vi "GaGe4_QueryStatus.vi"(8 "error in (no error)":errorcluster, 11 "Handle Cluster":T1) -> (0 "error out":errorcluster, 1 "Error?":bool, 2 "Triggered":bool, 4 "Complete":bool, 5 "Armed":bool, 6 "Status":string)   [LabVIEW 2015]
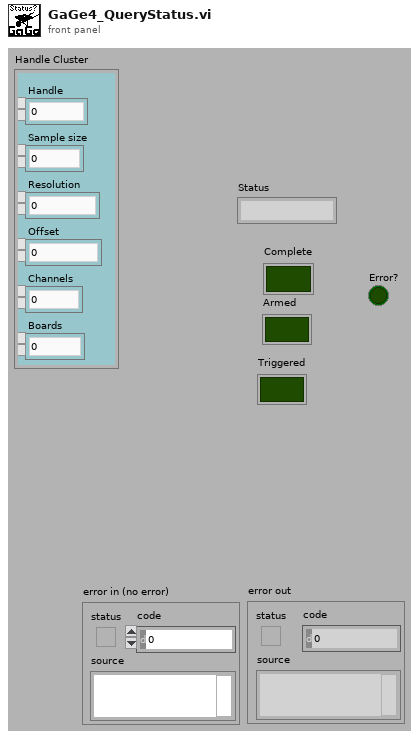
[diagram p1: front panel]
types:
  T1 = cluster{"Handle":u32, "Sample size":u32, "Resolution":i32, "Offset":i32, "Channels":u32, "Boards":u32}
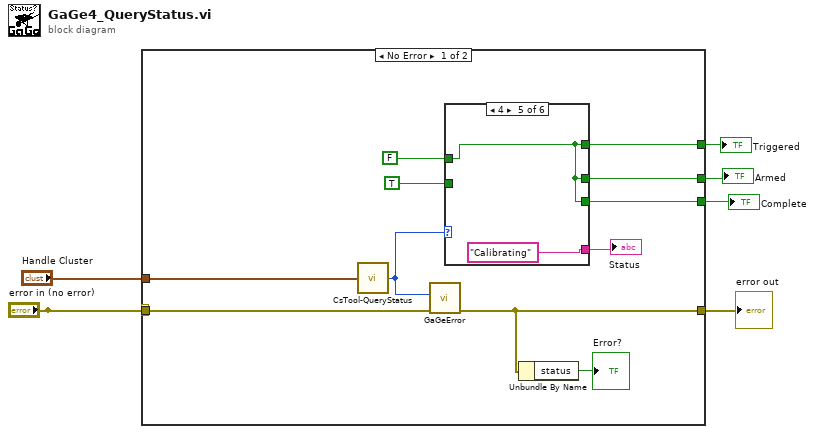
[diagram p0: block diagram]
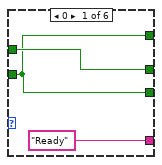
[diagram p2: hidden frame]
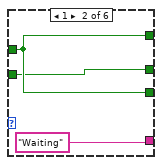
[diagram p3: hidden frame]
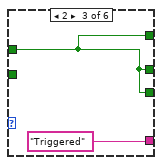
[diagram p4: hidden frame]
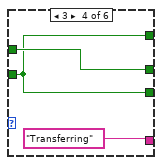
[diagram p5: hidden frame]
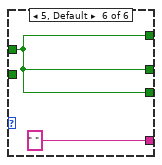
[diagram p6: hidden frame]
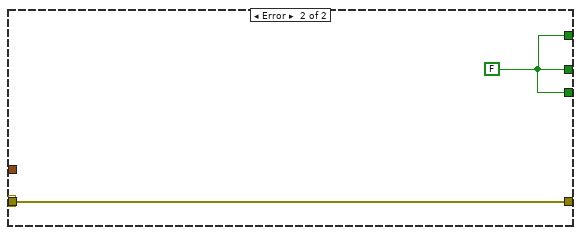
[diagram p7: hidden frame]
diagram:
  n1 = case shown="No Error" "error in (no error)" {
    tunnel: [w13 w33] -> w6
    tunnel: "Handle Cluster" -> [w7 _]
    tunnel: [w11 w34] -> w4
    tunnel: [w10 w34] -> w3
    tunnel: [w9 w34] -> w2
    tunnel: "error in (no error)" -> [w8 w33]
    frame No Error {
      n2 = call "CsTool-QueryStatus.vi"("Handle Cluster"=w7) -> ("Status"=w17:i32)
      n3 = call "GaGeError.vi"("error in (no error)"=w8, "Error Code"=w17) -> ("error out"=w13:errorcluster)  [unwired: 4 in, 5 out]
      n4 = case shown="4" w17 {
        tunnel: ["Ready" "Waiting" "Triggered" "Transferring" "Calibrating" " "] -> w14
        tunnel: FALSE -> [w19 w22 w24 w27 w29 w31]
        tunnel: TRUE -> [w18 w21 _ w26 _ _]
        tunnel: [w18 w22 w24 w26 w29 w31] -> w11
        tunnel: [w19 w21 w24 w27 w29 w31] -> w10
        tunnel: [w18 w22 w24 w26 w29 w31] -> w9
        frame 0 {
        }
        frame 1 {
        }
        frame 2 {
        }
        frame 3 {
        }
        frame 4 {
        }
        frame 5, Default {
        }
      }
      "Status" <- w14
      n5 = Unbundle By Name(w13) -> ("status"=→"Error?":bool)
    }
    frame Error {
      w34 = FALSE
    }
  }
  "error out" <- w6
  "Triggered" <- w2
  "Armed" <- w3
  "Complete" <- w4
